vi "Running Average Main Page.vi"(8 "error in (no error)":errorcluster, 11 "Node Ptr":T1 format="%.0x") -> (0 "error out":errorcluster)   [LabVIEW 2012, in "Running Average Custom Device.lvlib"]
uses:
  Running Average Custom Device.lvlib
  <vilib>/NI Veristand/Custom Device API/Custom Device Item Ref.ctl
  <vilib>/NI Veristand/Custom Device API/Custom Device Channel.ctl
  <vilib>/NI Veristand/Custom Device API/Custom Device Channel Type.ctl
  <vilib>/NI Veristand/Custom Device API/Get Item Property (U32).vi
  <vilib>/NI Veristand/Custom Device API/Get Item Property (String Array).vi
  <vilib>/NI Veristand/Custom Device API/Set Item Property (U32).vi
  <vilib>/NI Veristand/Custom Device API/Set Item Property (String Array).vi
  <vilib>/NI Veristand/Custom Device API/Custom Device API.lvlib
  <vilib>/NI Veristand/Custom Device Tools/Custom Device Utility Library/Custom Device Utility Library.lvlib
panel:
  in  "Channels Currently Added":i32(listbox)
  out "Channels":string[](array[string])
  in  "Configure Channels to Average":bool
  in  "Buffer Length":u32
  in  "Header":cluster{"Section Name":string}={"Section Name"="Custom Device Item Settings"}
  in  "Description":string
  in  "Name":string
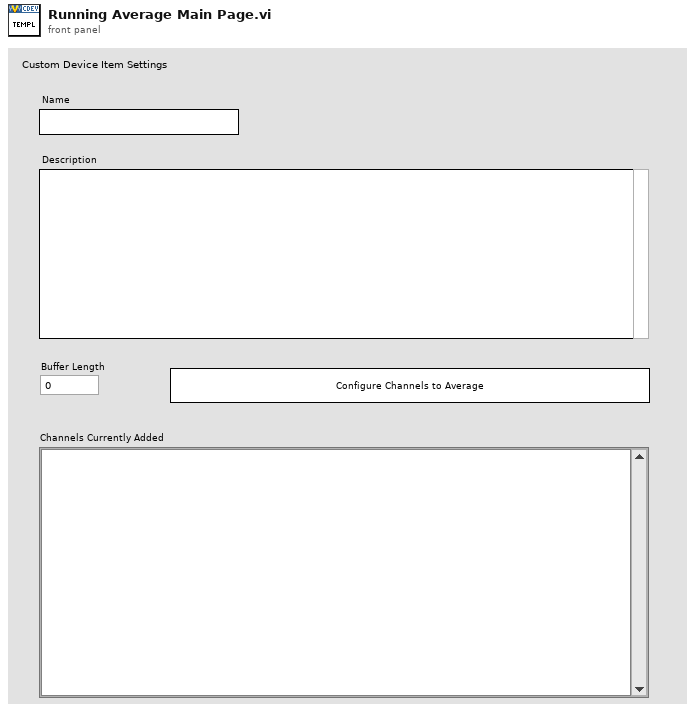
[diagram p1: front panel]
types:
  T1 = typedef "Custom Device API.lvlib/Custom Device Item Ref.ctl" = u64
  T2 = typedef "Custom Device API.lvlib/Custom Device Item Info.ctl" = cluster{"Name":string, "Is Channel":bool, "GUID":string, "Is Waveform":bool}
  T3 = typedef "Custom Device API.lvlib/Custom Device Channel.ctl" = cluster{"Type":T4, "Units":string, "Default Value":dbl, "Faultable":bool, "Scalable":bool}
  T4 = typedef "Custom Device API.lvlib/Custom Device Channel Type.ctl" = enum16{"Input", "Output"}
  T5 = typedef "Custom Device API.lvlib/Custom Device Commands.ctl" = enum16{"Default", "Item renamed", "Shutdown", "Dynamic button pressed"}
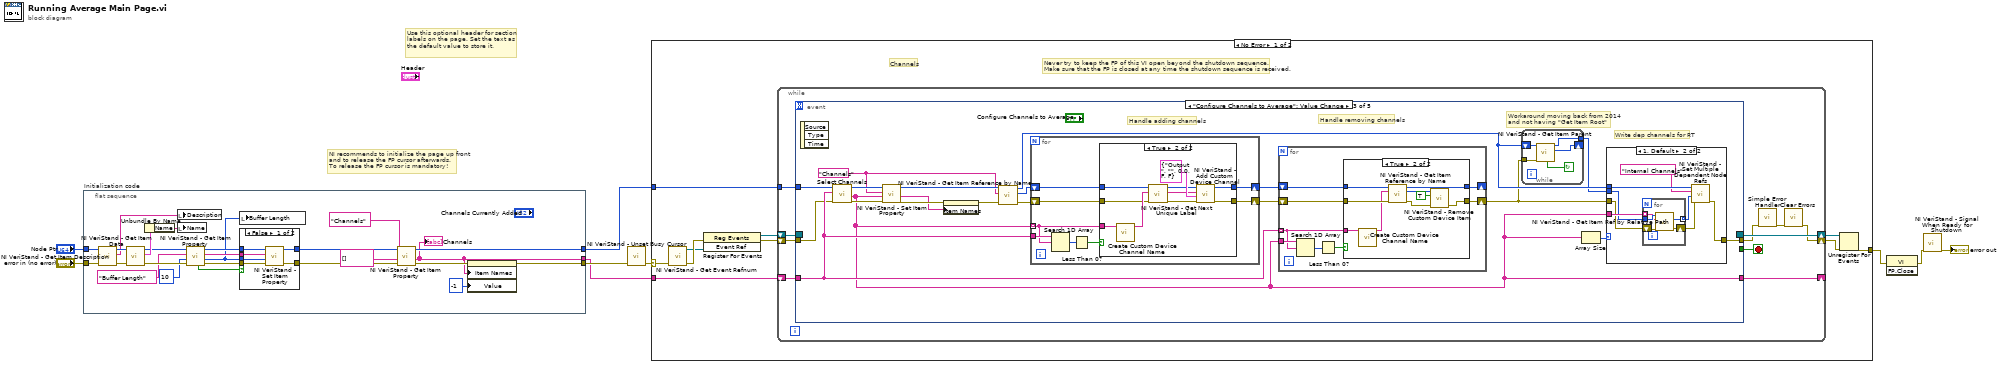
[diagram p0: block diagram]
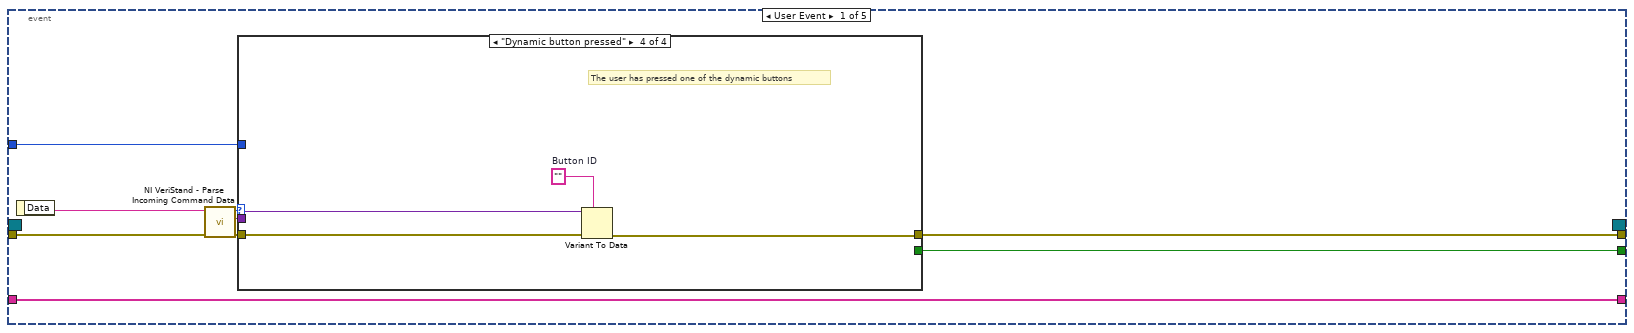
[diagram p2: hidden frame]
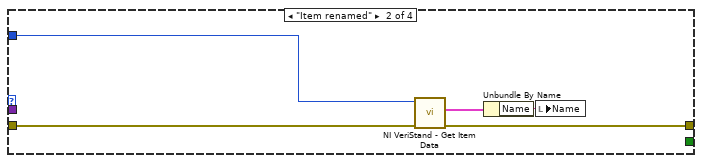
[diagram p4: hidden frame]
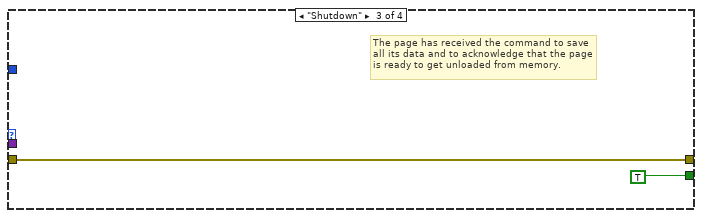
[diagram p5: hidden frame]
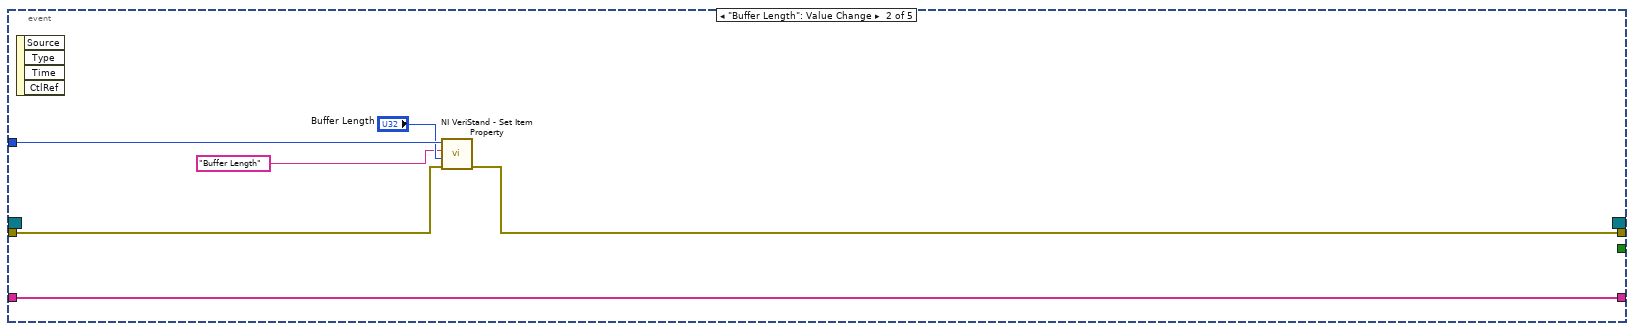
[diagram p6: hidden frame]
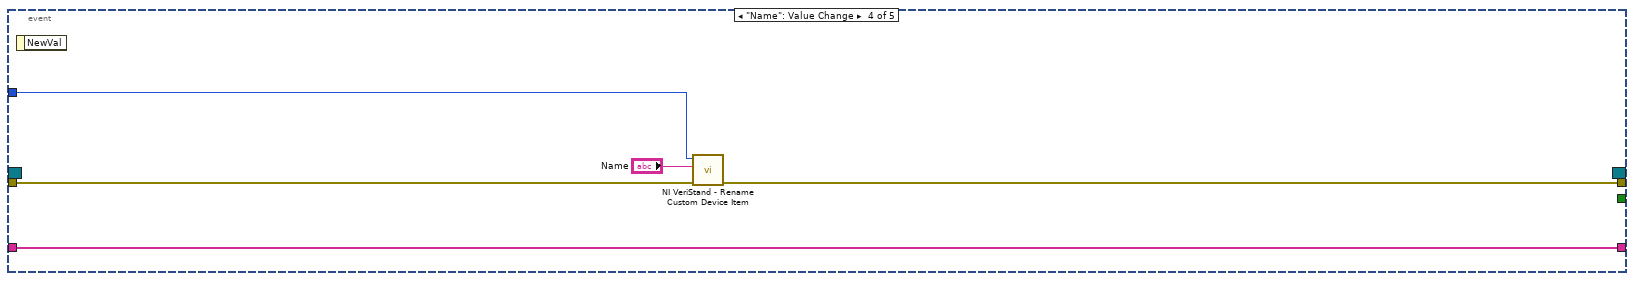
[diagram p10: hidden frame]
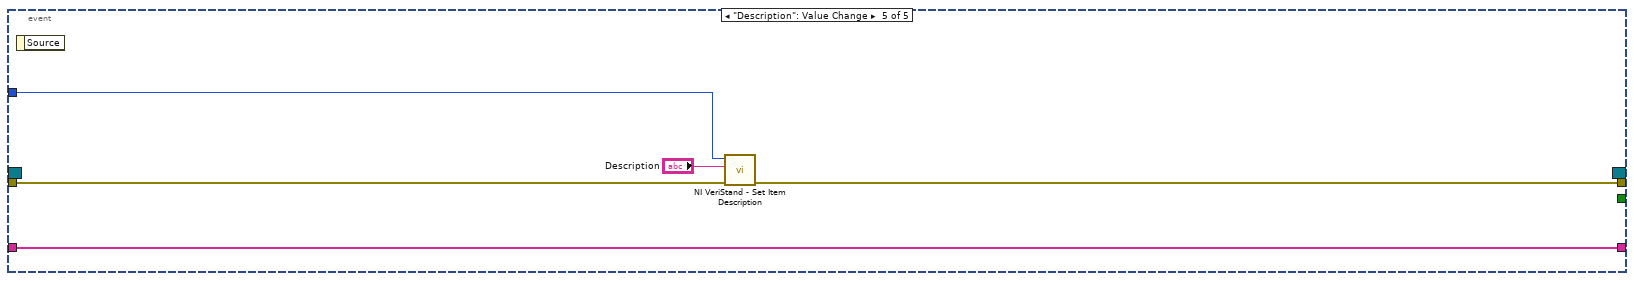
[diagram p11: hidden frame]
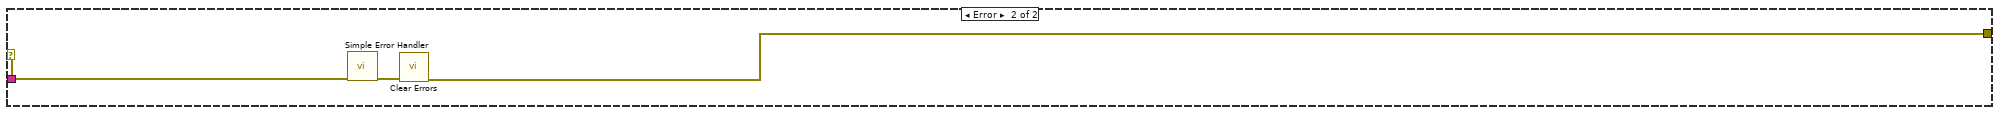
[diagram p12: hidden frame]
diagram:
  # "Use this optional header for section labels on the page. Set the text as the default value to store it."
  # "NI recommends to initialize the page up front\nand to release the FP cursor afterwards.\nTo release the FP cursor is mandatory!"
  n1 = flat-sequence "Initialization code" {
    tunnel: "error in (no error)" -> [w32]
    tunnel: "Node Ptr" -> [w21]
    tunnel: [w12] -> w5
    tunnel: [w24] -> w2
    tunnel: [w11] -> w1
    frame #0 {
      w15 = "Buffer Length" ("Property Name")
      n2 = call <vilib>:"NI VeriStand - Get Item Description.vi"("error in (no error)"=w32, "Item Ref in"=w21) -> ("error out"=w30:errorcluster, "Description"=w31:string, "Item Ref out"=w33:T1)  [unwired: 7 out]
      n3 = call <vilib>:"NI VeriStand - Get Item Data.vi"("error in (no error)"=w30, "Item Ref in"=w33) -> ("error out"=w27:errorcluster, "Item Info"=w29:T2, "Item Ref out"=w26:T1)  [unwired: 7 out]
      n4 = Unbundle By Name(w29) -> ("Name"=w28:string)
      n5 = local write "Description"(w31) -> ()
      n6 = local write "Name"(w28) -> ()
      n7 = call-poly <vilib>:"NI VeriStand - Get Item Property.vi"("error in (no error)"=w27, "Default Value"=u32 10, "Property Name"=w15, "Item Ref in"=w26) -> ("error out"=w18:errorcluster, "Value"=w14:u32, "Item Ref out"=w19:T1, "Found?"=w20:bool)  [unwired: 4 in]
      n8 = case shown="False" w20 {
        tunnel: w19 -> [w39 w41]
        tunnel: w18 -> [w38 w40]
        tunnel: [w35 w41] -> w17
        tunnel: [w34 w40] -> w16
        tunnel: w15 -> [w37 _]
        tunnel: w14 -> [w36 _]
        frame False {
          n9 = call-poly <vilib>:"NI VeriStand - Set Item Property.vi"("error in (no error)"=w38, "Value"=w36, "Property Name"=w37, "Item Ref in"=w39) -> ("error out"=w34:errorcluster, "Item Ref out"=w35:T1)  [unwired: 5 in, 1 out]
        }
        frame True {
        }
      }
      n10 = local write "Buffer Length"(w14) -> ()
      n11 = call-poly <vilib>:"NI VeriStand - Get Item Property.vi"("error in (no error)"=w16, "Default Value"=string[] [], "Property Name"="Channels", "Item Ref in"=w17) -> ("error out"=w13:errorcluster, "Value"=w11:string[], "Item Ref out"=w24:T1)  [unwired: 4 in, 1 out]
      "Channels" <- w11
      n12 = property on="Channels Currently Added" class="LstBox (strict)"(error in=w13, "Item Names"=w11, "Value"=-1 ("Channels Currently Added")) -> (error out=w12:errorcluster)  [unwired: 1 in, 1 out]
    }
  }
  n13 = call <vilib>:"NI VeriStand - Unset Busy Cursor.vi"("error in (no error)"=w5) -> ("error out"=w4:errorcluster)  [unwired: 10 out]
  n14 = case shown="No Error" w4 {
    selector: w4 -> [w43 w178]
    tunnel: [w48 w176] -> w9
    tunnel: w2 -> [w44 _]
    tunnel: w1 -> [w42 _]
    frame No Error {
      # "Channels"
      # "Never try to keep the FP of this VI open beyond the shutdown sequence.\nMake sure that the FP is closed at any time the shutdown sequence is received."
      n15 = call <vilib>:"NI VeriStand - Get Event Refnum.vi"("error in (no error)"=w43) -> ("error out"=w51:errorcluster, "Event Ref"=w47:refnum<user-event>)  [unwired: 9 out]
      n16 = register-events(error in=w51, w47) -> (reference out=w45:refnum<event-registration>, error out=w46:errorcluster)  [unwired: 1 in]
      n17 = while {
        tunnel: w44 -> [w57]
        shift-right: [w54] -> w49
        shift-left: w46 -> [w60]
        shift-right: [w61] -> w50
        shift-left: w45 -> [w59]
        shift-right: [w52] -> _
        shift-left: w42 -> [w53]
        stop <- w58 stop-if-true
        n18 = event shown="[2] \"Configure Channels to Average\": Value Change" {
          selector: w59 -> [_ _ _ _ _]
          dyn-events: [_ _ _ _ _] -> w61
          timeout: _ -> [_ _ _ _ _]
          tunnel: w60 -> [w70 w85 w100 w170 w174]
          tunnel: [w66 _ _ _ _] -> w58
          tunnel: [w65 w84 w105 w169 w173] -> w56
          tunnel: w57 -> [w64 w88 w103 w168 w175]
          tunnel: w53 -> [w62 w83 w102 w166 w171]
          tunnel: [w62 w83 w96 w166 w171] -> w52
          event User Event {
            n19 = event-data() -> ("Data"=w69:string)  [unwired: 1 out]
            n20 = call <vilib>:"NI VeriStand - Parse Incoming Command Data.vi"("error in (no error)"=w70, "Incoming data"=w69) -> ("error out"=w68:errorcluster, "Outgoing data"=w63:variant, "Action"=w67:T5)  [unwired: 7 out]
            n21 = case shown="\"Dynamic button pressed\"" w67 {
              tunnel: w68 -> [w71 w76 w77 w82]
              tunnel: [_ _ TRUE _] -> w66
              tunnel: [w71 w73 w77 w79] -> w65
              tunnel: w64 -> [_ w75 _ _]
              tunnel: w63 -> [_ _ _ w81]
              frame "Default", Default {
              }
              frame "Item renamed" {
                n22 = call <vilib>:"NI VeriStand - Get Item Data.vi"("error in (no error)"=w76, "Item Ref in"=w75) -> ("error out"=w73:errorcluster, "Item Info"=w74:T2)  [unwired: 8 out]
                n23 = Unbundle By Name(w74) -> ("Name"=w72:string)
                n24 = local write "Name"(w72) -> ()
              }
              frame "Shutdown" {
                # "The page has received the command to save all its data and to acknowledge that the page is ready to get unloaded from memory."
              }
              frame "Dynamic button pressed" {
                w80 = ""  # Button ID
                # "The user has pressed one of the dynamic buttons"
                n25 = Variant To Data(error in=w82, type=w80, Variant=w81) -> (error out=w79:errorcluster)  [unwired: 1 out]
              }
            }
          }
          event "Buffer Length": Value Change {
            n26 = event-data() -> ()  [unwired: 5 out]
            n27 = call-poly <vilib>:"NI VeriStand - Set Item Property.vi"("error in (no error)"=w85, "Value"="Buffer Length", "Property Name"="Buffer Length", "Item Ref in"=w88) -> ("error out"=w84:errorcluster)  [unwired: 5 in, 2 out]
          }
          event "Configure Channels to Average": Value Change {
            w92 = "Channels" ("Property Name")
            # "Workaround moving back from 2014\nand not having \"Get Item Root\""
            # "Write dep channels for RT"
            # "Handle removing channels"
            # "Handle adding channels"
            n28 = event-data() -> ()  [unwired: 4 out]
            n29 = call "Select Channels.vi"("error in (no error)"=w100, "Channels to Highlight"=w102, "Item Ref In"=w103) -> ("error out"=w99:errorcluster, "Channels Selected"=w96:string[], "Dup Item Ref"=w101:T1)  [unwired: 6 in]
            n30 = call-poly <vilib>:"NI VeriStand - Set Item Property.vi"("error in (no error)"=w99, "Value"=w96, "Property Name"=w92, "Item Ref in"=w101) -> ("error out"=w98:errorcluster, "Item Ref out"=w94:T1)  [unwired: 5 in, 1 out]
            n31 = property on="Channels Currently Added" class="LstBox (strict)"(error in=w98, "Item Names"=w96) -> (error out=w97:errorcluster)  [unwired: 1 in, 1 out]
            n32 = call <vilib>:"NI VeriStand - Get Item Reference by Name.vi"("error in (no error)"=w97, "Item Name"=w92, "Parent Ref in"=w94) -> ("error out"=w95:errorcluster, "Item Ref"=w93:T1, "Parent Ref out"=w91:T1)  [unwired: 5 in, 1 out]
            n33 = for {
              tunnel: w96 -> [w149] mode=indexing
              tunnel: w102 -> [w153]
              shift-right: [w148] -> w106
              shift-left: w95 -> [w150]
              shift-right: [w146] -> w107
              shift-left: w93 -> [w147]
              n34 = Search 1D Array(1D array=w153, element=w149) -> (index of element=w152:i32)  [unwired: 1 in]
              n35 = Less Than 0?(x=w152) -> (x < 0?=w151:bool)
              n36 = case shown="True" w151 {
                tunnel: w147 -> [w154 w163]
                tunnel: w150 -> [w155 w161]
                tunnel: w149 -> [_ w158]
                tunnel: [w155 w156] -> w148
                tunnel: [w154 w157] -> w146
                frame False {
                }
                frame True {
                  n37 = call "Create Custom Device Channel Name.vi"("Channel Path"=w158) -> ("CD Name"=w164:string)  [unwired: 10 in]
                  n38 = call <vilib>:"NI VeriStand - Get Next Unique Label.vi"("error in (no error)"=w161, "Label"=w164, "Parent Ref in"=w163) -> ("error out"=w160:errorcluster, "Label out"=w162:string, "Parent Ref dup"=w159:T1)  [unwired: 5 in, 1 out]
                  n39 = call <vilib>:"NI VeriStand - Add Custom Device Channel.vi"("error in (no error)"=w160, "Channel"=T3 {"Type"=enum."Output", "Units"="", "Default Value"=0.0, "Faultable"=FALSE, "Scalable"=FALSE}, "Channel Name"=w162, "Parent Ref in"=w159) -> ("error out"=w156:errorcluster, "Parent Ref out"=w157:T1)  [unwired: 4 in, 2 out]
                }
              }
            }
            n40 = for {
              tunnel: w102 -> [w131] mode=indexing
              tunnel: w96 -> [w134]
              shift-right: [w129] -> w90
              shift-left: w106 -> [w130]
              shift-right: [w127] -> _
              shift-left: w107 -> [w128]
              n41 = Search 1D Array(1D array=w134, element=w131) -> (index of element=w133:i32)  [unwired: 1 in]
              n42 = Less Than 0?(x=w133) -> (x < 0?=w132:bool)
              n43 = case shown="True" w132 {
                tunnel: w131 -> [_ w139]
                tunnel: w128 -> [w135 w144]
                tunnel: w130 -> [w136 w143]
                tunnel: [w136 w140] -> w129
                tunnel: [w135 w137] -> w127
                frame False {
                }
                frame True {
                  n44 = call "Create Custom Device Channel Name.vi"("Channel Path"=w139) -> ("CD Name"=w138:string)  [unwired: 10 in]
                  n45 = call <vilib>:"NI VeriStand - Get Item Reference by Name.vi"("error in (no error)"=w143, "Item Name"=w138, "Parent Ref in"=w144) -> ("error out"=w141:errorcluster, "Item Ref"=w142:T1, "Parent Ref out"=w137:T1)  [unwired: 5 in, 1 out]
                  n46 = call <vilib>:"NI VeriStand - Remove Custom Device Item.vi"("error in (no error)"=w141, "Force Delete (F)"=TRUE, "Item Ref in"=w142) -> ("error out"=w140:errorcluster)  [unwired: 7 in, 1 out]
                }
              }
            }
            n47 = while {
              shift-right: [w109] -> _
              shift-left: w91 -> [w112]
              tunnel: w90 -> [w111]
              tunnel: [w110] -> w89
              stop <- w108 continue-if-true
              n48 = call <vilib>:"NI VeriStand - Get Item Parent.vi"("error in (no error)"=w111, "Item Ref in"=w112) -> ("Parent Ref"=w109:T1, "Item Ref out"=w110:T1, "Found"=w108:bool)  [unwired: 6 in, 1 out]
            }
            n49 = Array Size(array=w96) -> (size(s)=w104:i32)
            n50 = case shown="1, Default" w104 {
              tunnel: w96 -> [_ w121]
              tunnel: w91 -> [_ w120]
              tunnel: [w113 w118] -> w105
              tunnel: w90 -> [w113 w117]
              tunnel: w89 -> [_ w114]
              frame 0 {
              }
              frame 1, Default {
                n51 = for {
                  tunnel: w121 -> [w125] mode=indexing
                  tunnel: [w122] -> w115 mode=indexing
                  shift-right: [w123] -> w116
                  shift-left: w117 -> [w124]
                  tunnel: w114 -> [w126]
                  n52 = call <vilib>:"NI VeriStand - Get Item Ref by Relative Path.vi"("error in"=w124, "Relative Item Path"=w125, "Section Ref in"=w126) -> ("error out"=w123:errorcluster, "Item Ref"=w122:T1)  [unwired: 5 in, 2 out]
                }
                n53 = call <vilib>:"NI VeriStand - Set Multiple Dependent Node Refs.vi"("error in (no error)"=w116, "Dependent Node Refs"=w115, "Base Property Name"="Internal Channels", "Item Ref in"=w120) -> ("error out"=w118:errorcluster)  [unwired: 6 in, 1 out]
              }
            }
          }
          event "Name": Value Change {
            n54 = event-data() -> ()  [unwired: 2 out]
            n55 = call <vilib>:"NI VeriStand - Rename Custom Device Item.vi"("error in (no error)"=w170, "New Name"="Name", "Item Ref in"=w168) -> ("error out"=w169:errorcluster)  [unwired: 1 in, 7 out]
          }
          event "Description": Value Change {
            n56 = event-data() -> ()  [unwired: 2 out]
            n57 = call <vilib>:"NI VeriStand - Set Item Description.vi"("error in (no error)"=w174, "Description"="Description", "Item Ref in"=w175) -> ("error out"=w173:errorcluster)  [unwired: 8 out]
          }
        }
        n58 = call <vilib>:"Simple Error Handler.vi"("error in (no error)"=w56) -> ("error out"=w55:errorcluster)  [unwired: 1 in, 7 out]
        n59 = call <vilib>:"Clear Errors.vi"("error in (no error)"=w55) -> ("error out"=w54:errorcluster)  [unwired: 6 out]
      }
      n60 = Unregister For Events(event registration refnum=w50, error in=w49) -> (error out=w48:errorcluster)
    }
    frame Error {
      n61 = call <vilib>:"Simple Error Handler.vi"("error in (no error)"=w178) -> ("error out"=w177:errorcluster)  [unwired: 1 in, 7 out]
      n62 = call <vilib>:"Clear Errors.vi"("error in (no error)"=w177) -> ("error out"=w176:errorcluster)  [unwired: 6 out]
    }
  }
  n63 = invoke class="VI" method="FP.Close"(error in=w9) -> (error out=w8:errorcluster)  [unwired: 2 in, 2 out]
  n64 = call <vilib>:"NI VeriStand - Signal When Ready for Shutdown.vi"("error in (no error)"=w8) -> ("error out"=→"error out":errorcluster)  [unwired: 10 out]
